vi "GetPos.vi"(6 "Position 2":refnum<vi>, 8 "error in (no error)":errorcluster, 11 "Rele in":refnum<class "Rele.lvclass">) -> (0 "error out":errorcluster, 2 "Position":dbl, 3 "Rele out":refnum<class "Rele.lvclass">)   [LabVIEW 2012, in "Rele.lvclass"]
uses:
  Rele.lvclass
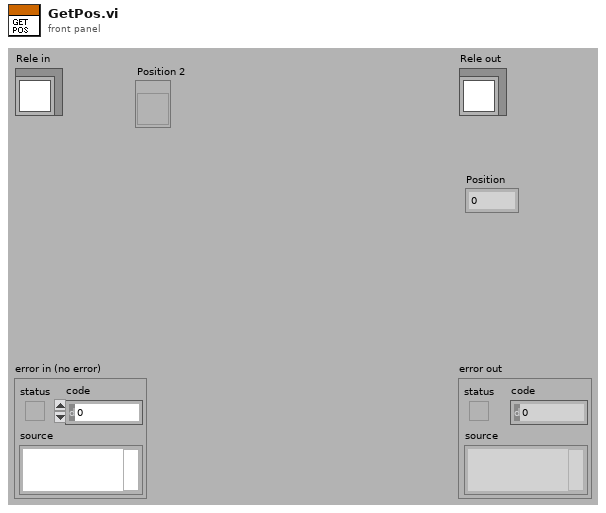
[diagram p1: front panel]
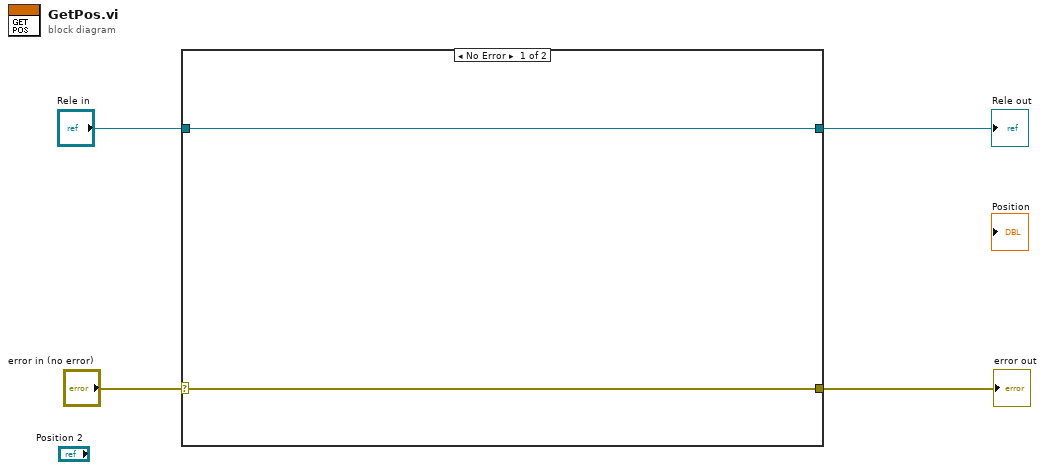
[diagram p0: block diagram]
diagram:
  n1 = case shown="No Error" "error in (no error)" {
    selector: "error in (no error)" -> [w5 w7]
    tunnel: "Rele in" -> [w6 w8]
    tunnel: [w6 w8] -> w2
    tunnel: [w5 w7] -> w1
    frame No Error {
    }
    frame Error {
    }
  }
  "error out" <- w1
  "Rele out" <- w2
